vi "利用SQL语句访问数据库 - 副本.vi"(0 "参数配置":T2={"connection reference"=refnum, "数据库名称"="", "TABLE"="", "模拟运行"=FALSE, "数据库操作"=enum."DELETE", "error in (no error)"={"status"=FALSE, "code"=0, "source"=""}}, 1 "附件条件":bool, 2 "附加语句":string, 3 "one column data":string[](array[string]), 4 "Insert Data":string[](array[string])=["5", "D", "5", "2015/1/19 14:41:15"], 5 "columns":string[](array[string]), 6 "待操作的列名":string, 7 "待操作的列名对应的数据":string) -> (14 "connection reference 2":T1, 18 "数据":string[][](array[string]), 19 "error out":errorcluster)   [LabVIEW 2014]
uses:
  <vilib>/addons/database/Connection.llb/Conn ObjectReference.ctl
  <vilib>/addons/database/Connection.llb/DB Tools Open Connec (String).vi
  <vilib>/addons/database/Connection.llb/Conn Execute.vi
  <vilib>/addons/database/Recordset.llb/Rec Fetch Recordset Data (R).vi
  <vilib>/addons/database/Recordset.llb/Rec Destroy - Connection.vi
  <vilib>/addons/database/NI_Database_API.lvlib
panel:
  # "UPDATE"
  # "one column data:\n                        列名1\n                        列名1数据\n                        需要操作的列的列名\n                         需要操作的列的数据"
  # "SELECT"
  # "DELETE"
  # "主键不能用单引号,更新多个数据\n时，在第一项中输入列名1='',\n列名2='',......列名n，第二项中输入\n列名n对应的数据"
  # "INSERT"
  # "两者数组大小必须保持一样的"
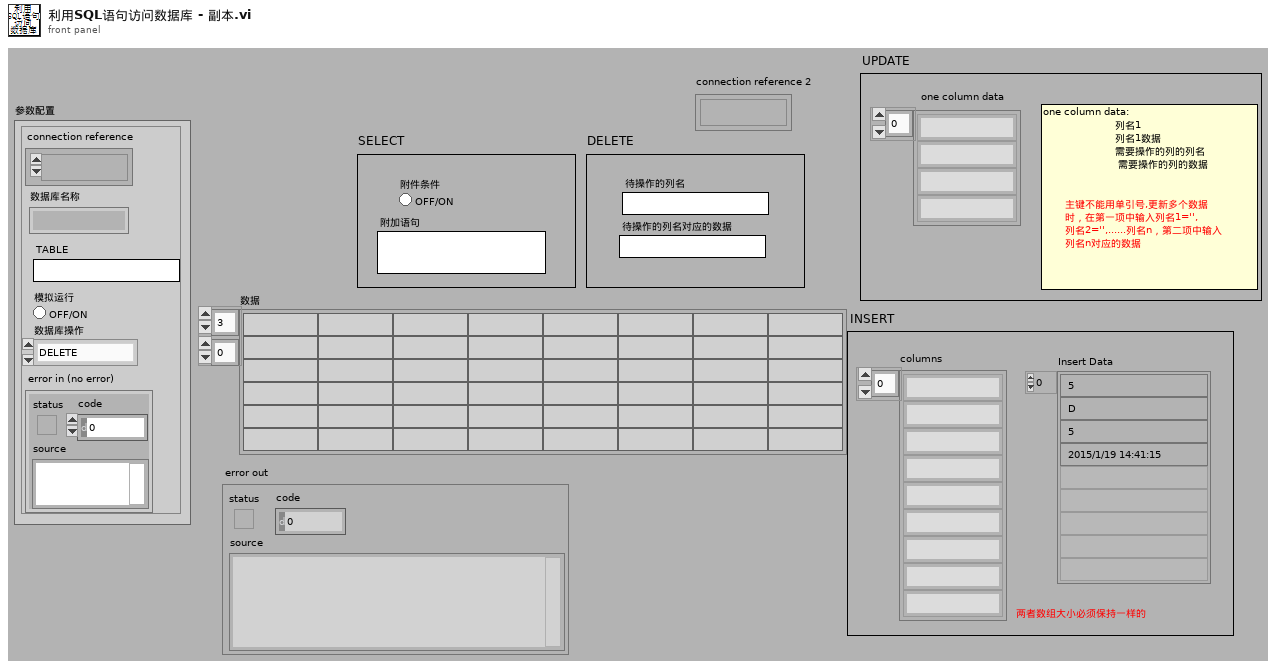
[diagram p1: front panel]
types:
  T1 = typedef "NI_Database_API.lvlib/Conn ObjectReference.ctl" = refnum<k1>
  T2 = cluster{"connection reference":T1, "数据库名称":string, "TABLE":string, "模拟运行":bool, "数据库操作":enum16{"SELECT", "UPDATE", "INSERT", "DELETE"}, "error in (no error)":errorcluster}
  T3 = typedef "NI_Database_API.lvlib/Rec ObjectReference.ctl" = refnum<k1>
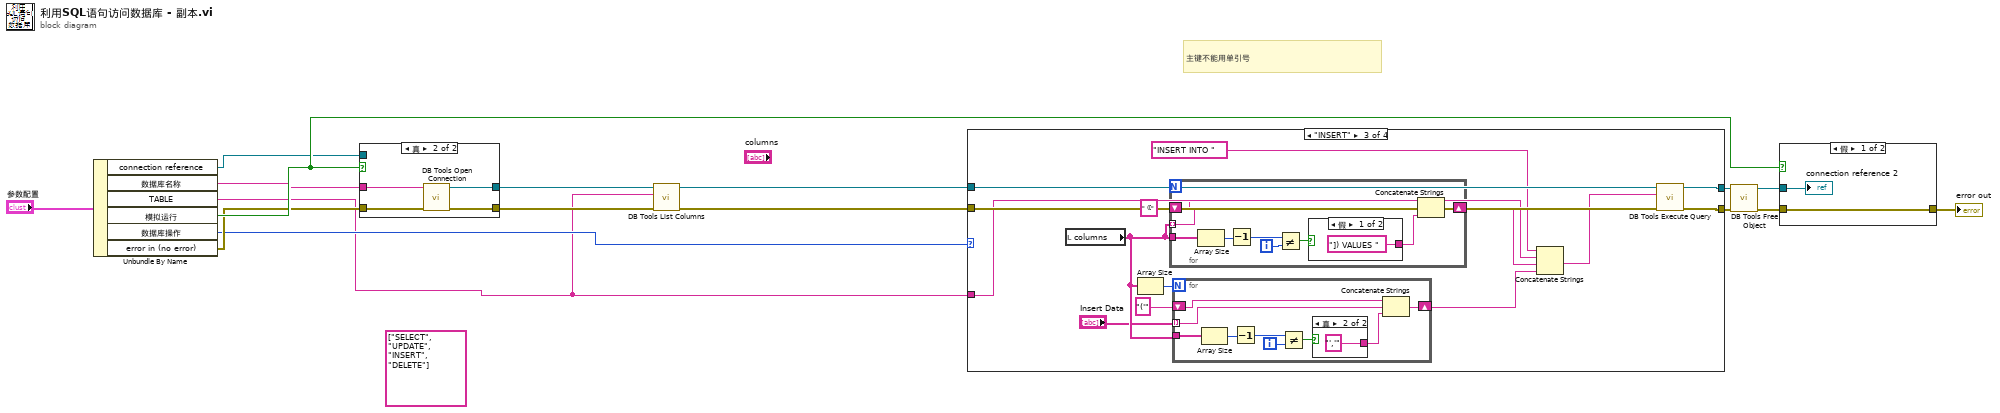
[diagram p0: block diagram]
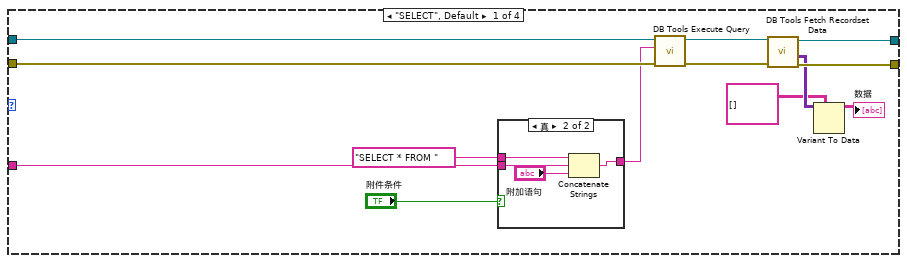
[diagram p2: hidden frame]
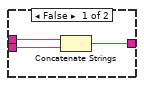
[diagram p3: hidden frame]
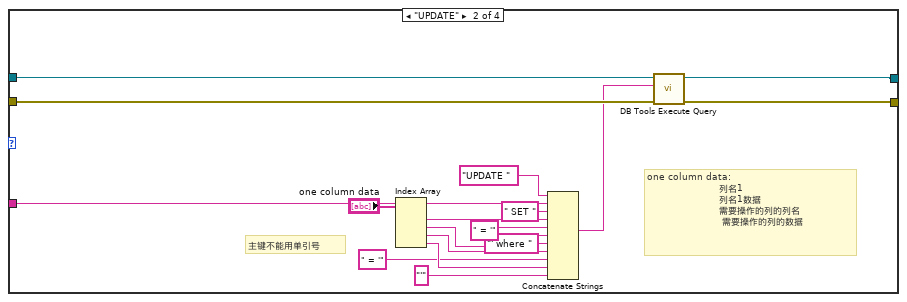
[diagram p4: hidden frame]
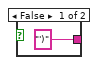
[diagram p5: hidden frame]
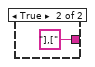
[diagram p6: hidden frame]
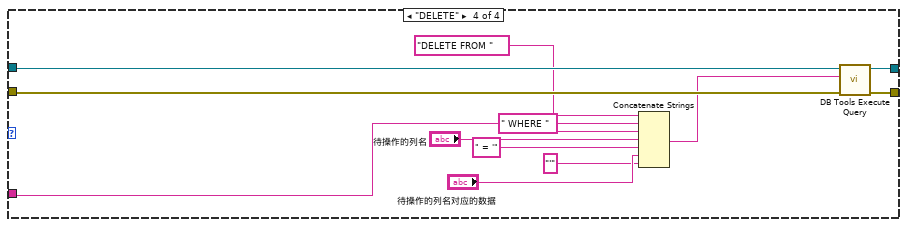
[diagram p7: hidden frame]
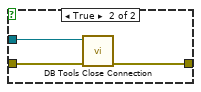
[diagram p8: hidden frame]
diagram:
  (unwired) string[] ["SELECT", "UPDATE", "INSERT", "DELETE"]
  # "主键不能用单引号"
  n1 = Unbundle By Name("参数配置") -> ("connection reference"=w1:T1, "数据库名称"=w2:string, "TABLE"=w3:string, "模拟运行"=w6:bool, "数据库操作"=w4:enum16{"SELECT", "UPDATE", "INSERT", "DELETE"}, "error in (no error)"=w5:errorcluster)
  n2 = case shown="真" w6 {
    tunnel: [w17 w22] -> w11
    tunnel: w5 -> [w18 w21]
    tunnel: [w18 w20] -> w10
    tunnel: w2 -> [_ w19]
    tunnel: w1 -> [w17 _]
    frame False {
    }
    frame True {
      n3 = call-poly <vilib>:"DB Tools Open Connection.vi"("error in (no error)"=w21, "connection information"=w19) -> ("error out"=w20:errorcluster, "connection reference"=w22:T1)  [unwired: 6 in]
    }
  }
  n4 = call <vilib>:"DB Tools List Columns.vi"("error in (no error)"=w10, "table"=w3, "connection reference"=w11) -> ("error out"=w8:errorcluster, "connection reference out"=w9:T1)  [unwired: 1 in, 2 out]
  n5 = case shown="\"INSERT\"" w4 {
    tunnel: [w33 w46 w71 w107] -> w16
    tunnel: [w32 w45 w70 w106] -> w15
    tunnel: w9 -> [w31 w49 w73 w105]
    tunnel: w8 -> [w30 w48 w72 w104]
    tunnel: w3 -> [w23 w57 w61 w102]
    frame "SELECT", Default {
      n6 = case shown="真" "附件条件" {
        tunnel: "SELECT * FROM " ("字符串") -> [w38 w42]
        tunnel: [w36 w40] -> w24
        tunnel: w23 -> [w37 w39]
        frame False {
          n7 = Concatenate Strings(w38, w37) -> (w36:string)
        }
        frame True {
          n8 = Concatenate Strings(w42, w39, "附加语句") -> (w40:string)
        }
      }
      n9 = call-poly <vilib>:"DB Tools Execute Query.vi"("error in (no error)"=w30, "SQL query"=w24, "connection reference"=w31) -> ("error out"=w34:errorcluster, "recordset reference"=w35:T3)  [unwired: 5 in]
      n10 = call-poly <vilib>:"DB Tools Fetch Recordset Data.vi"("error in (no error)"=w34, "recordset reference"=w35) -> ("error out"=w32:errorcluster, "recordset data"=w29:variant[][], "recordset reference out"=w33:T3)  [unwired: 3 in]
      n11 = Variant To Data(type=string[][] [], Variant=w29) -> (data=→"数据":string[][])  [unwired: 1 in, 1 out]
    }
    frame "UPDATE" {
      # "主键不能用单引号"
      # "one column data:\n                        列名1\n                        列名1数据\n                        需要操作的列的列名\n                         需要操作的列的数据"
      n12 = Index Array(array="one column data") -> (element #1=w55:string, element #2=w54:string, element #3=w52:string, element #4=w50:string)  [unwired: 4 in]
      n13 = Concatenate Strings("UPDATE ", w57, " SET " ("字符串"), w55, " = '" ("字符串"), w54, "' where " ("字符串"), w52, " = '" ("字符串"), w50, "'" ("字符串")) -> (w47:string)
      n14 = call-poly <vilib>:"DB Tools Execute Query.vi"("error in (no error)"=w48, "SQL query"=w47, "connection reference"=w49) -> ("error out"=w45:errorcluster, "recordset reference"=w46:T3)  [unwired: 5 in]
    }
    frame "INSERT" {
      n15 = local read "columns"() -> (w68:string[])
      n16 = Array Size(array=w68) -> (size(s)=w67:i32)
      n17 = for {
        tunnel: w68 -> [w93] mode=indexing
        shift-right: [w92] -> w65
        shift-left: " ([" -> [w91]
        tunnel: w68 -> [w89]
        i -> [w86]
        n18 = Array Size(array=w89) -> (size(s)=w88:i32)
        n19 = Decrement(x=w88) -> (x-1=w87:i32)
        n20 = Not Equal?(x=w87, y=w86) -> (x != y?=w85:bool)
        n21 = case shown="假" w85 {
          tunnel: ["]) VALUES " ("字符串") "],[" ("字符串")] -> w90
          frame False {
          }
          frame True {
          }
        }
        n22 = Concatenate Strings(w91, w93, w90) -> (w92:string)
      }
      n23 = for {
        N: w67 -> [_]
        tunnel: "Insert Data" -> [w82] mode=indexing
        shift-right: [w81] -> w66
        shift-left: "('" -> [w80]
        tunnel: w68 -> [w78]
        i -> [w75]
        n24 = Array Size(array=w78) -> (size(s)=w77:i32)
        n25 = Decrement(x=w77) -> (x-1=w76:i32)
        n26 = Not Equal?(x=w76, y=w75) -> (x != y?=w74:bool)
        n27 = case shown="真" w74 {
          tunnel: ["')" ("字符串") "','" ("字符串")] -> w79
          frame False {
          }
          frame True {
          }
        }
        n28 = Concatenate Strings(w80, w82, w79) -> (w81:string)
      }
      n29 = Concatenate Strings("INSERT INTO ", w61, w65, w66) -> (w60:string)
      n30 = call-poly <vilib>:"DB Tools Execute Query.vi"("error in (no error)"=w72, "SQL query"=w60, "connection reference"=w73) -> ("error out"=w70:errorcluster, "recordset reference"=w71:T3)  [unwired: 5 in]
    }
    frame "DELETE" {
      n31 = Concatenate Strings("DELETE FROM " ("字符串"), w102, " WHERE " ("字符串"), "待操作的列名", " = '" ("字符串"), "待操作的列名对应的数据", "'" ("字符串")) -> (w97:string)
      n32 = call-poly <vilib>:"DB Tools Execute Query.vi"("error in (no error)"=w104, "SQL query"=w97, "connection reference"=w105) -> ("error out"=w106:errorcluster, "recordset reference"=w107:T3)  [unwired: 5 in]
    }
  }
  n33 = call-poly <vilib>:"DB Tools Free Object.vi"("error in (no error)"=w15, "recordset reference"=w16) -> ("error out"=w13:errorcluster, "connection reference"=w14:T1)  [unwired: 8 in]
  n34 = case shown="假" w6 {
    tunnel: w14 -> [w109 w112]
    tunnel: w13 -> [w108 w111]
    tunnel: [w108 w110] -> w12
    frame False {
      "connection reference 2" <- w109
    }
    frame True {
      n35 = call <vilib>:"DB Tools Close Connection.vi"("error in (no error)"=w111, "connection reference"=w112) -> ("error out"=w110:errorcluster)  [unwired: 5 in]
    }
  }
  "error out" <- w12
